vi "divide_checker.vi"(11 "H_lk":ext[][](array[numeric])) -> (3 "H_lk":ext[][](array[numeric]))   [LabVIEW 2013]
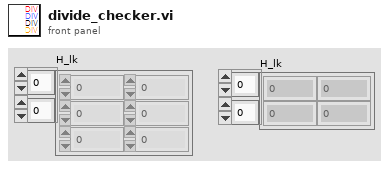
[diagram p1: front panel]
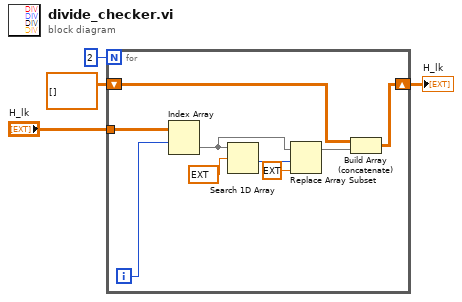
[diagram p0: block diagram]
diagram:
  n1 = for {
    N: 2 -> [_]
    tunnel: "H_lk" -> [w13]
    shift-right: [w6] -> w1
    shift-left: ext[][] [] -> [w5]
    i -> [w12]
    n2 = Index Array(array=w13, index (row)=w12) -> (element=w10:ext[])  [unwired: 1 in]
    n3 = Search 1D Array(1D array=w10, element=ext nan) -> (index of element=w9:i32)  [unwired: 1 in]
    n4 = Replace Array Subset(array=w10, new element=ext 0.0 ("new element/subarray"), index=w9) -> (w7:ext[])
    n5 = Build Array (concatenate)(w5, w7) -> (w6:ext[][])
  }
  "H_lk" <- w1
